vi "Obtain Control Cluster.vi"(9 "I/O":bool=TRUE, 11 "Motion":bool=TRUE) -> (3 "Control Out":T1)   [LabVIEW 2016, in "Controller.lvclass"]
uses:
  Controller.lvclass
  Controllers.ctl
  Motion/Copy of Motion Folder/Motion.lvclass
  I-O/Copy of I-O Folder/I-O.lvclass
  Dispenser/Copy of Dispenser Folder/Dispenser.lvclass
  Motion/Copy of A3200 Folder/A3200.lvclass
  D:/INTT/Classes/Controllers/Motion/Copy of Motion Folder/Motion.lvclass
  I-O/Copy of NI-DAQ Folder/NI-DAQ.lvclass
  D:/INTT/Classes/Controllers/I-O/Copy of I-O Folder/I-O.lvclass
  Dispenser/Copy of Ultimus V2 Folder/Ultimus V2.lvclass
  D:/INTT/Classes/Controllers/Dispenser/Copy of Dispenser Folder/Dispenser.lvclass
panel:
  in  "Dispense":bool
  in  "Control":T1
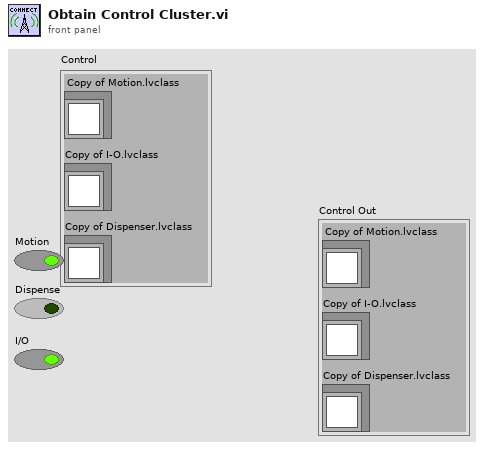
[diagram p1: front panel]
types:
  T1 = typedef "Controller.lvclass/Controllers.ctl" = cluster{"Copy of Motion.lvclass":refnum<class "Motion.lvclass">, "Copy of I-O.lvclass":refnum<class "I-O.lvclass">, "Copy of Dispenser.lvclass":refnum<class "Dispenser.lvclass">}
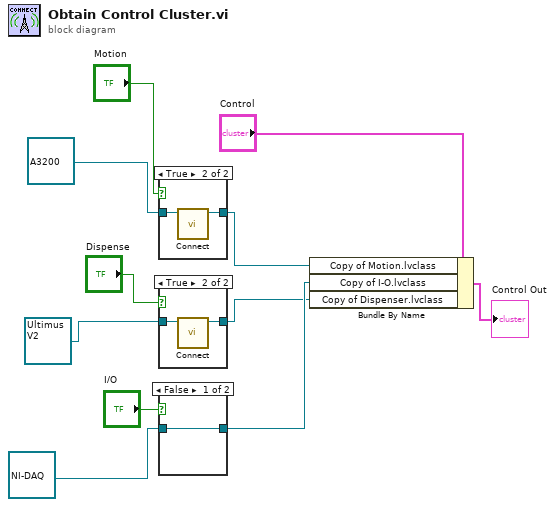
[diagram p0: block diagram]
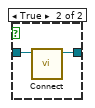
[diagram p4: hidden frame]
diagram:
  n1 = case shown="True" "Motion" {
    tunnel: [w12 w13] -> w5
    tunnel: refnum<class "A3200.lvclass"> refnum ("Copy of A3200.lvclass") -> [w12 w14]
    frame False {
    }
    frame True {
      n2 = call-dynamic "Connect.vi"("Gantry in"=w14) -> ("Gantry out"=w13:refnum<class "A3200.lvclass">)  [unwired: 9 in, 1 out]
    }
  }
  n3 = case shown="True" "Dispense" {
    tunnel: refnum<class "Ultimus V2.lvclass"> refnum ("Copy of Ultimus V2.lvclass") -> [w15 w17]
    tunnel: [w15 w16] -> w1
    frame False {
    }
    frame True {
      n4 = call-dynamic "Connect.vi"("Ultimus V in"=w17) -> ("Ultimus V out"=w16:refnum<class "Ultimus V2.lvclass">)  [unwired: 9 in, 1 out]
    }
  }
  n5 = case shown="False" "I/O" {
    tunnel: refnum<class "NI-DAQ.lvclass"> refnum ("Copy of NI-DAQ.lvclass") -> [w18 w20]
    tunnel: [w18 w19] -> w4
    frame False {
    }
    frame True {
      n6 = call-dynamic "Connect.vi"("NI-DAQ in"=w20) -> ("NI-DAQ out"=w19:refnum<class "NI-DAQ.lvclass">)  [unwired: 9 in, 1 out]
    }
  }
  n7 = Bundle By Name(cluster="Control", "Copy of Motion.lvclass"=w5, "Copy of I-O.lvclass"=w4, "Copy of Dispenser.lvclass"=w1) -> (→"Control Out":T1)
